vi "Create Probabilistic_OccupancyGrid.vi"(8 "error in (no error)":errorcluster, 10 "occupancy grid":dbl[][](array[numeric])) -> (0 "error out":errorcluster, 3 "Probabilistic_OccupancyGrid out":refnum<class "Probabilistic_OccupancyGrid.lvclass">)   [LabVIEW 2017, in "Probabilistic_OccupancyGrid.lvclass"]
uses:
  Probabilistic_OccupancyGrid.lvclass
  Probabilistic_OccupancyGrid.lvclass/Probabilistic_OccupancyGrid.ctl
  <vilib>/robotics/Utilities/NI_Robotics Utilities.lvlib
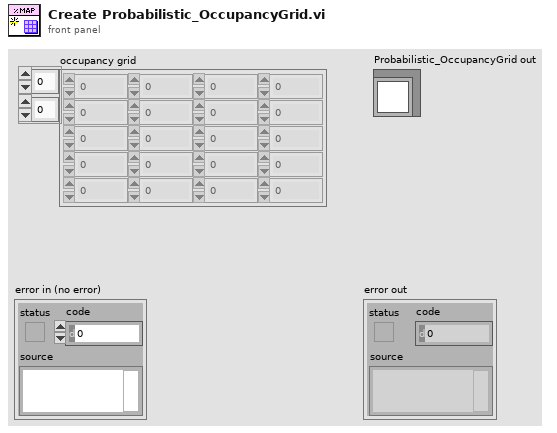
[diagram p1: front panel]
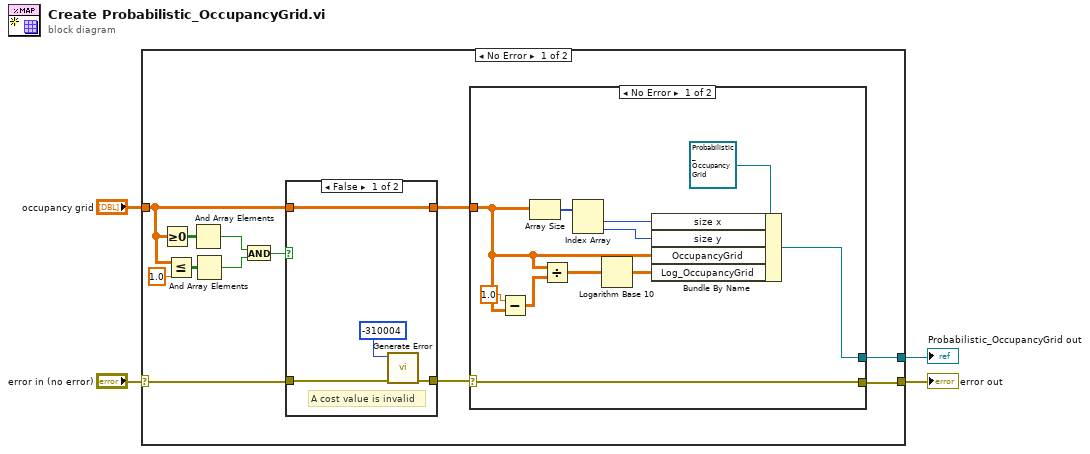
[diagram p0: block diagram]
diagram:
  n1 = case shown="No Error" "error in (no error)" {
    selector: "error in (no error)" -> [w13 w35]
    tunnel: [w15 w35] -> w2
    tunnel: "occupancy grid" -> [w10 _]
    tunnel: [w16 _] -> w1
    frame No Error {
      n2 = Greater Or Equal To 0?(x=w10) -> (x >= 0?=w14:bool[][])
      n3 = Less Or Equal?(x=w10, y=1.0) -> (x <= y?=w8:bool[][])
      n4 = And Array Elements(Boolean array=w14) -> (logical AND=w7:bool)
      n5 = And Array Elements(Boolean array=w8) -> (logical AND=w6:bool)
      n6 = And(x=w7, y=w6) -> (x .and. y?=w5:bool)
      n7 = case shown="False" w5 {
        tunnel: [w19 w22] -> w12
        tunnel: w13 -> [w20 w22]
        tunnel: [w18 w21] -> w11
        tunnel: w10 -> [w18 w21]
        frame False {
          # "A cost value is invalid"
          n8 = call <vilib>:"Generate Error.vi"("error in (no error)"=w20, "code"=-310004) -> ("error out"=w19:errorcluster)  [unwired: 9 in]
        }
        frame True {
        }
      }
      n9 = case shown="No Error" w12 {
        selector: w12 -> [w30 w34]
        tunnel: [w28 _] -> w16
        tunnel: [w30 w34] -> w15
        tunnel: w11 -> [w25 _]
        frame No Error {
          n10 = Subtract(x=1.0, y=w25) -> (x-y=w24:dbl[][])
          n11 = Array Size(array=w25) -> (size(s)=w33:i32[])
          n12 = Divide(x=w25, y=w24) -> (x/y=w23:dbl[][])
          n13 = Index Array(array=w33) -> (element #1=w32:i32, element #2=w31:i32)  [unwired: 2 in]
          n14 = Logarithm Base 10(1:w23) -> (0:w27:dbl[][])
          n15 = Bundle By Name(cluster=refnum<class "Probabilistic_OccupancyGrid.lvclass"> refnum ("Probabilistic_OccupancyGrid out"), "size x"=w32, "size y"=w31, "OccupancyGrid"=w25, "Log_OccupancyGrid"=w27) -> (w28:refnum<class "Probabilistic_OccupancyGrid.lvclass">)
        }
        frame Error {
        }
      }
    }
    frame Error {
    }
  }
  "Probabilistic_OccupancyGrid out" <- w1
  "error out" <- w2
